vi "limitron.vi"(5 "Encoder Value from Playback":dbl, 9 "Playback Active":bool, 11 "Hardware In":cluster{"Motor Name":string, "EncoderDevRef":T1}={"Motor Name"="", "EncoderDevRef"={"DevStatus"={"status"=FALSE, "code"=0, "source"=""}, "EncoderIndex"=enum."Invalid", "CounterIndex"=enum."Invalid", "DistancePerCount"=1.0, "Decoding Type"=enum."4x"}}) -> (2 "Allow Drive":bool, 3 "Taper Control":dbl)   [LabVIEW 2017]
uses:
  <vilib>/Rock Robotics/WPI/Encoder/WPI_EncoderDevRef.ctl
  <vilib>/Rock Robotics/SystemInterfaces/Encoder/FPGA_EncoderIdx.ctl
  <vilib>/Rock Robotics/SystemInterfaces/Counter/FPGA_CounterCtrSystemIndex.ctl
  <vilib>/Rock Robotics/WPI/Encoder/WPI_EncoderType.ctl
  <vilib>/addons/control/pid/pid.llb/PID (DBL).vi
  globals.vi
  <vilib>/addons/control/pid/NI_PID_pid.lvlib
panel:
  out "match timer":bool
  in  "PID gains":T5={"proportional gain (Kc)"=1.0, "integral time (Ti, min)"=0.01, "derivative time (Td, min)"=0.0} {"derivative time (Td, min)" format="%.3f"; "integral time (Ti, min)" format="%.3f"; "proportional gain (Kc)" format="%.3f"}
  in  "Clockwise":bool
  in  "Taper Maximum":dbl
  in  "Discretionary Setpoint":dbl
  in  "Taper Limit":dbl
  in  "Discretionary Limit":dbl
  # "The Taper Control is the output to the Playback function.\nIt messages the playback function to limit the max PID \noutput when the arm is past the Taper Limit"
  # "Allow Drive prevents drive when the Recorded Value taken \nfrom playback is not on the correct side of the Discretionary Setpoint"
  # "NOTE: NOT SURE WHICH IS WHICH, DOUBLE CHECK"
  # "Past this point, forces playback.vi\nto slow down"
  # "Discretionary Limit. Limitron BEGINS to use PID and forces playback.vi to yield control."
  # "Discretionary Setpoint. Limitron attempts to hold this by\nforcing playback.vi to yield control, and holding this position with PID"
  # "This is a Hard Limit, ARM MUST NOT PASS THIS POINT.\nLimitron uses the motors to enforce this fact."
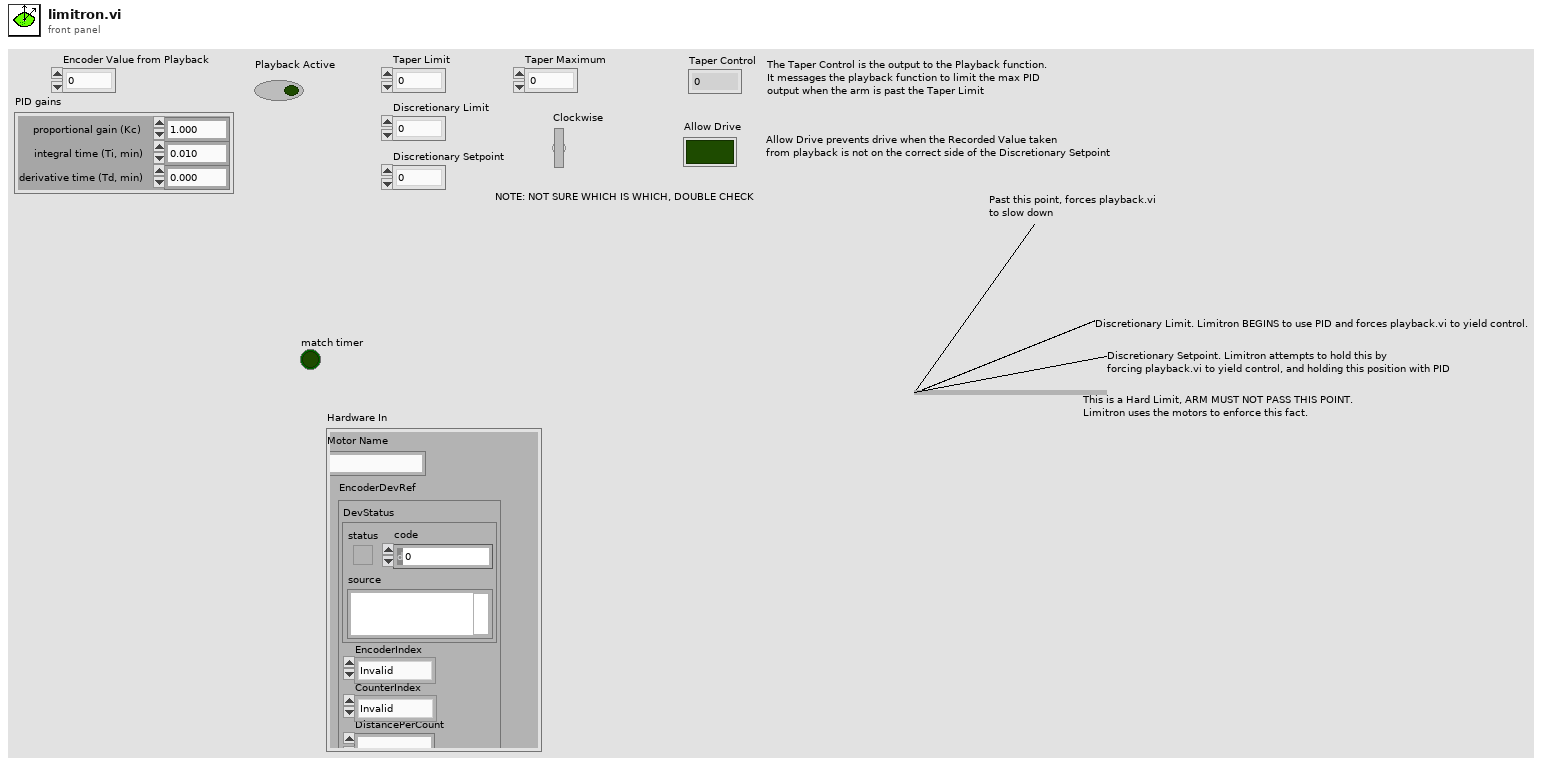
[diagram p1: front panel]
types:
  T1 = typedef "WPI_EncoderDevRef.ctl" = cluster{"DevStatus":errorcluster, "EncoderIndex":T2, "CounterIndex":T3, "DistancePerCount":dbl, "Decoding Type":T4}
  T2 = typedef "FPGA_EncoderIdx.ctl" = enum8{"Enc 0", "Enc 1", "Enc 2", "Enc 3", "Enc 4", "Enc 5", "Enc 6", "Enc 7", "Invalid"}
  T3 = typedef "FPGA_CounterCtrSystemIndex.ctl" = enum8{"Ctr 0", "Ctr 1", "Ctr 2", "Ctr 3", "Ctr 4", "Ctr 5", "Ctr 6", "Ctr 7", "Invalid"}
  T4 = typedef "WPI_EncoderType.ctl" = enum16{"1x", "2x", "4x"}
  T5 = cluster{"proportional gain (Kc)":dbl, "integral time (Ti, min)":dbl, "derivative time (Td, min)":dbl}
  T6 = typedef "WPI_MotorControlDeviceRef.ctl" = cluster{"DeviceStatus":errorcluster, "Type":T7, "PWM":cluster{"PWM Channel":T8, "DeadBand":T9}, "CAN":cluster{"Device Number":u8, "SetOutput VI Ref":variant, "GetOutput VI Ref":variant, "Enable VI Ref":variant, "Disable VI Ref":variant, "Data":variant}, "Invert":bool, "DIO PWM":cluster{"PWM \"Enable\" Channel":T8, "DIOChannel":T10, "PWM Rate":dbl}}
  T7 = typedef "WPI_MotorControlType.ctl" = enum16{"PWM", "CAN", "DIO PWM"}
  T8 = typedef "FPGA_DIOPWMChannel.ctl" = enum8{"PWM 0", "PWM 1", "PWM 2", "PWM 3", "PWM 4", "PWM 5", "PWM 6", "PWM 7", "PWM 8", "PWM 9", "PWM MXP 0", "PWM MXP 1", "PWM MXP 2", "PWM MXP 3", "PWM MXP 4", "PWM MXP 5", "PWM MXP 6", "PWM MXP 7", "PWM MXP 8", "PWM MXP 9", "Invalid"}
  T9 = typedef "WPI_PWMDeadband.ctl" = cluster{"Name":string, "maxPositivePwm":i32, "minPositivePwm":i32, "centerPwm":i32, "maxNegativePwm":i32, "minNegativePwm":i32, "angularRange":u16}
  T10 = typedef "FPGA_DIOChannel.ctl" = enum8{"DIO 0", "DIO 1", "DIO 2", "DIO 3", "DIO 4", "DIO 5", "DIO 6", "DIO 7", "DIO 8", "DIO 9", "DIO MXP 0", "DIO MXP 1", "DIO MXP 2", "DIO MXP 3", "DIO MXP 4", "DIO MXP 5", "DIO MXP 6", "DIO MXP 7", "DIO MXP 8", "DIO MXP 9", "DIO MXP 10", "DIO MXP 11", "DIO MXP 12", "DIO MXP 13", "DIO MXP 14", "DIO MXP 15", "SPI Port CS1", "SPI Port CS2", "SPI Port CS3", "SPI Port MISO", "SPI Port MOSI", "Invalid"}
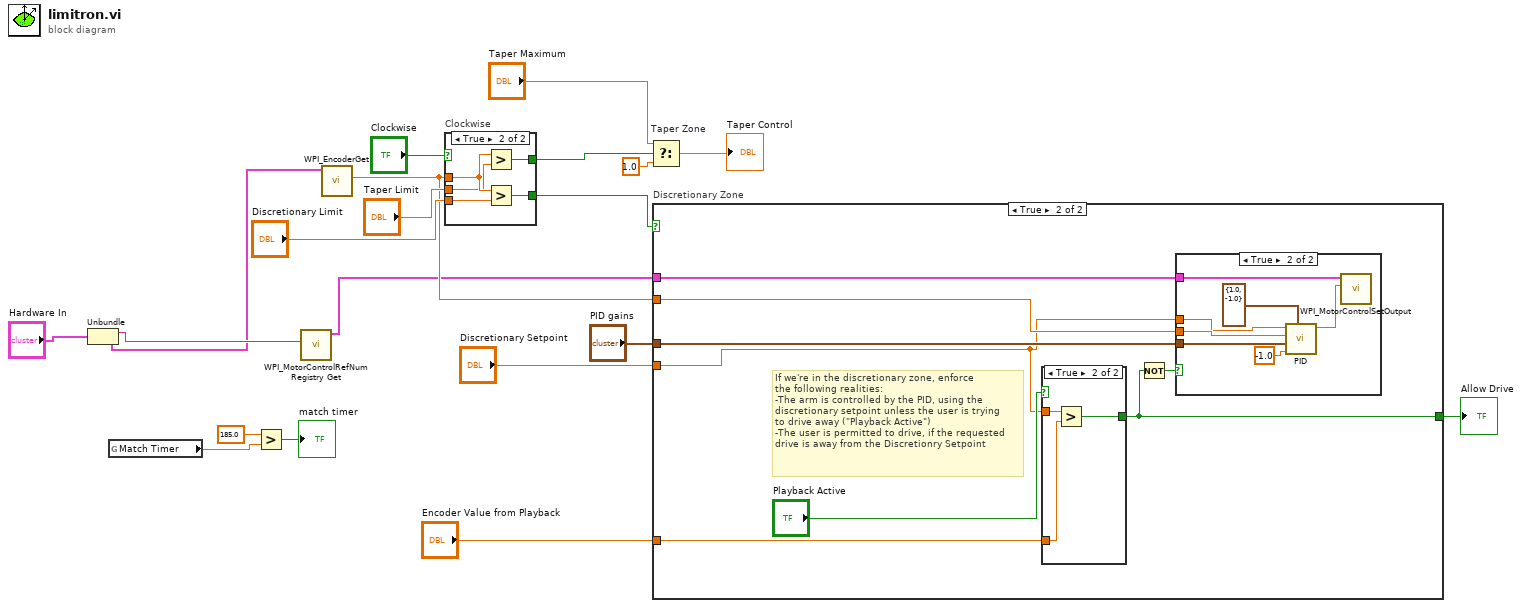
[diagram p0: block diagram]
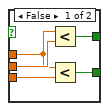
[diagram p2: hidden frame]
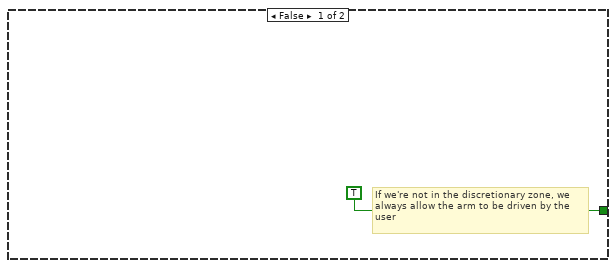
[diagram p3: hidden frame]
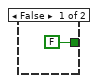
[diagram p5: hidden frame]
diagram:
  n1 = Unbundle("Hardware In") -> ("Motor Name"=w2:string, "EncoderDevRef"=w1:T1)
  n2 = global read "globals.vi" "Match Timer"() -> (w6:dbl)
  n3 = Greater?(x=185.0, y=w6) -> (0:→"match timer":bool)
  n4 = call <vilib>:"WPI_MotorControlRefNum Registry Get.vi"("refnum name"=w2) -> ("MotorControlDevRef"=w4:T6)  [unwired: 9 in, 1 out]
  n5 = call <vilib>:"WPI_EncoderGet.vi"("EncoderDevRef"=w1) -> ("Distance"=w10:dbl)  [unwired: 5 in, 5 out]
  n6 = case "Clockwise" shown="True" "Clockwise" {
    tunnel: w10 -> [w23 w30]
    tunnel: "Taper Limit" -> [w24 w29]
    tunnel: [w25 w28] -> w16
    tunnel: [w21 w27] -> w15
    tunnel: "Discretionary Limit" -> [w22 w26]
    frame False {
      n7 = Less?(x=w23, y=w24) -> (x < y?=w25:bool)
      n8 = Less?(x=w23, y=w22) -> (x < y?=w21:bool)
    }
    frame True {
      n9 = Greater?(x=w30, y=w29) -> (0:w28:bool)
      n10 = Greater?(x=w30, y=w26) -> (0:w27:bool)
    }
  }
  n11 = Select "Taper Zone"(t="Taper Maximum", s=w16, f=1.0) -> (s? t:f=→"Taper Control":dbl)
  n12 = case "Discretionary Zone" shown="True" w15 {
    tunnel: [TRUE ("Allow Drive") w34] -> w12
    tunnel: "Discretionary Setpoint" -> [_ w35]
    tunnel: w10 -> [_ w39]
    tunnel: "PID gains" -> [_ w38]
    tunnel: "Encoder Value from Playback" -> [_ w36]
    tunnel: w4 -> [_ w32]
    frame False {
      # "If we're not in the discretionary zone, we\nalways allow the arm to be driven by the\nuser"
    }
    frame True {
      # "If we're in the discretionary zone, enforce\nthe following realities:\n-The arm is controlled by the PID, using the\ndiscretionary setpoint unless the user is trying\nto drive away (\"Playback Active\")\n-The user is permitted to drive, if the requested\ndrive is away from the Discretionry Setpoint"
      n13 = case shown="True" "Playback Active" {
        tunnel: [FALSE w48] -> w34
        tunnel: w36 -> [_ w49]
        tunnel: w35 -> [_ w50]
        frame False {
        }
        frame True {
          n14 = Greater?(x=w50, y=w49) -> (0:w48:bool)
        }
      }
      n15 = Not(x=w34) -> (.not. x?=w33:bool)
      n16 = case shown="True" w33 {
        tunnel: w39 -> [_ w46]
        tunnel: w38 -> [_ w44]
        tunnel: w32 -> [_ w41]
        tunnel: w35 -> [_ w40]
        frame False {
        }
        frame True {
          n17 = call-poly <vilib>:"PID.vi"("output range"=cluster{"output high":dbl, "output low":dbl} {"output high"=1.0, "output low"=-1.0}, "dt (s)"=-1.0, "PID gains"=w44, "process variable"=w46, "setpoint"=w40) -> ("output"=w42:dbl)  [unwired: 5 in, 1 out]
          n18 = call <vilib>:"WPI_MotorControlSetOutput.vi"("Output"=w42, "MotorControlDevRef"=w41) -> ()  [unwired: 7 in, 3 out]
        }
      }
    }
  }
  "Allow Drive" <- w12
